vi "E7_20_READ_BUFFER.vi"(8 "error in":T6, 11 "DriverConnect in":T1={"InterfaceType"=enum."VISA", "OpenedSession"="", "InterfaceSettings"={"Interface"=enum."RS232", "EOS 4 read"=enum."LF (\\n)", "EOS 4 write"=enum."LF (\\n)", "TMO, ms"=10000, "Sett"=variant(cluster{"Baud Rate":u32, "Data Bits":u16, "Parity":u16, "Stop Bits":u16, "Flow Control":u16, "Eho":bool} {"Baud Rate"=75, "Data Bits"=0, "Parity"=0, "Stop Bits"=0, "Flow Control"=0, "Eho"=FALSE})}}) -> (0 "error out":T6, 3 "DriverConnect out":T1={"InterfaceType"=enum."VISA", "OpenedSession"="", "InterfaceSettings"={"Interface"=enum."RS232", "EOS 4 read"=enum."LF (\\n)", "EOS 4 write"=enum."LF (\\n)", "TMO, ms"=10000, "Sett"=variant(cluster{"Baud Rate":u32, "Data Bits":u16, "Parity":u16, "Stop Bits":u16, "Flow Control":u16, "Eho":bool} {"Baud Rate"=75, "Data Bits"=0, "Parity"=0, "Stop Bits"=0, "Flow Control"=0, "Eho"=FALSE})}}, 5 "String":string)   [LabVIEW 2018]
uses:
  MOKO_LabViewLibrary/MokoLowLevel/MokoLowLovelControl/MLLC_Error.ctl
  MOKO_LabViewLibrary/MokoLowLevel/MokoLowLovelControl/MLLC_ConnectCluster.ctl
  MOKO_LabViewLibrary/MokoLowLevel/MokoLowLovelControl/MLLC_InterfaceType.ctl
  MOKO_LabViewLibrary/MokoLowLevel/MokoLowLovelControl/MLLC_OpenedSession.ctl
  MOKO_LabViewLibrary/MokoLowLevel/MokoLowLovelControl/MLLC_InterfaceSettings.ctl
  MOKO_LabViewLibrary/MokoLowLevel/MokoLowLovelControl/MLLC_InterfaceKind.ctl
  MOKO_LabViewLibrary/MokoLowLevel/MokoLowLovelControl/MLLC_Rs232Settings.ctl
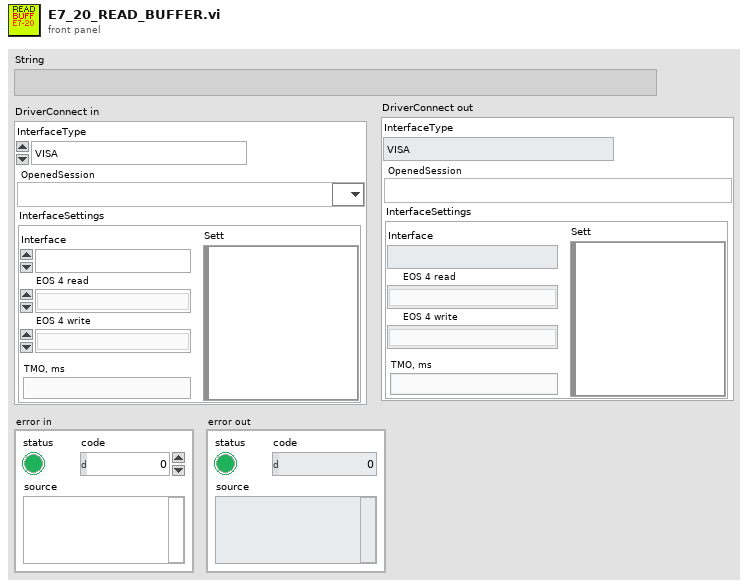
[diagram p1: front panel]
types:
  T1 = typedef "MLLC_ConnectCluster.ctl" = cluster{"InterfaceType":T2, "OpenedSession":T3, "InterfaceSettings":T4}
  T2 = typedef "MLLC_InterfaceType.ctl" = enum16{"VISA", "Prologix USB-GPIB"}
  T3 = typedef "MLLC_OpenedSession.ctl" = refnum<visa-resource-name>
  T4 = typedef "MLLC_InterfaceSettings.ctl" = cluster{"Interface":T5, "EOS 4 read":enum16{"Default (=EOS 4 write)", "CR (\\r)", "LF (\\n)", "None"}, "EOS 4 write":enum16{"CR+LF (\\r\\n)", "CR (\\r)", "LF (\\n)", "None"}, "TMO, ms":i32, "Sett":variant}
  T5 = typedef "MLLC_InterfaceKind.ctl" = enum16{"RS232", "GPIB", "USB", "Ethernet", "another"}
  T6 = typedef "MLLC_Error.ctl" = errorcluster
  T7 = typedef "MLLC_Rs232Settings.ctl" = cluster{"Baud Rate":u32, "Data Bits":u16, "Parity":u16, "Stop Bits":u16, "Flow Control":u16, "Eho":bool}
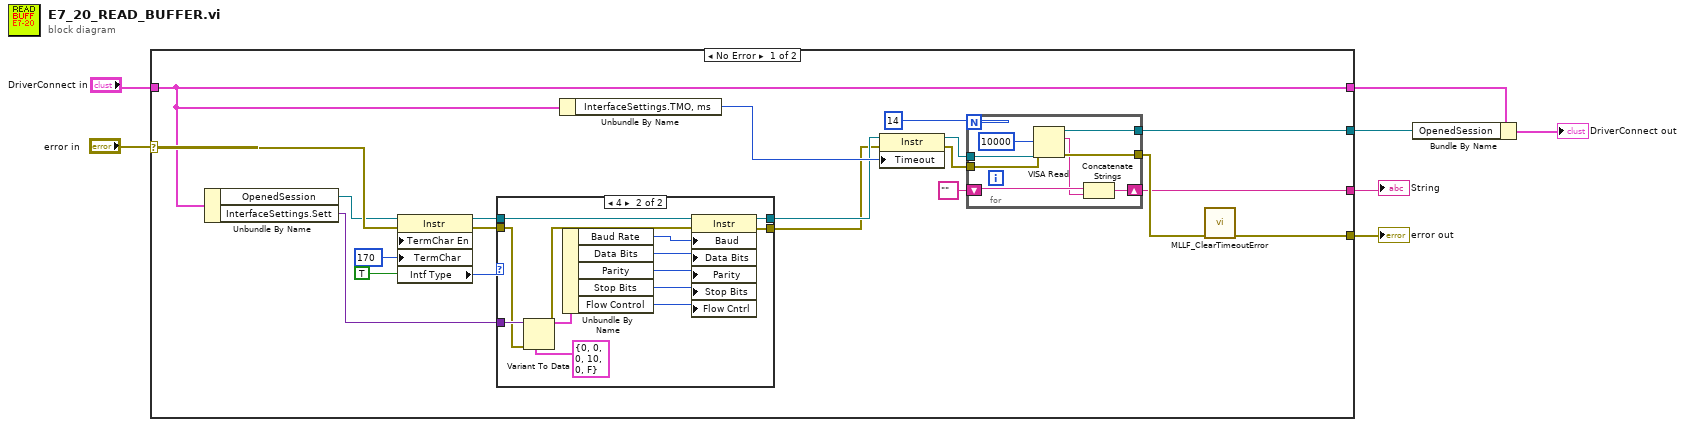
[diagram p0: block diagram]
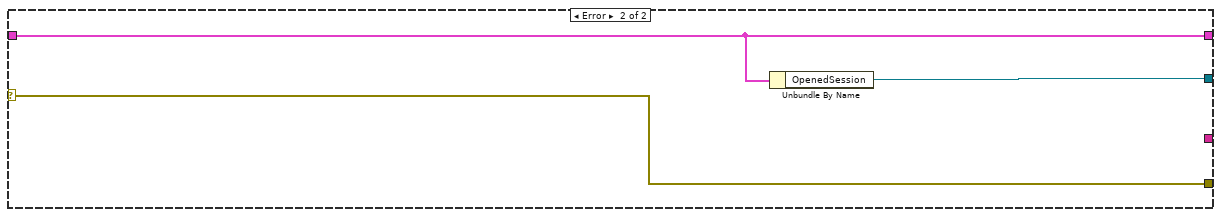
[diagram p3: hidden frame]
diagram:
  n1 = case shown="No Error" "error in" {
    selector: "error in" -> [w25 w53]
    tunnel: [w13 _] -> w7
    tunnel: [w27 w53] -> w6
    tunnel: [w14 w51] -> w3
    tunnel: [w9 w52] -> w2
    tunnel: "DriverConnect in" -> [w9 w52]
    frame No Error {
      n2 = Unbundle By Name(w9) -> ("OpenedSession"=w8:T3, "InterfaceSettings.Sett"=w22:variant)
      n3 = property class="Instr"(reference=w8, error in=w25, "TermChar En"=TRUE ("Message Based Settings:Termination Character Enable"), "TermChar"=u16 170 ("Message Based Settings:Termination Character")) -> (reference out=w24:T3, error out=w23:errorcluster, "Intf Type"=w18:u16)
      n4 = case shown="4" w18 {
        tunnel: [w37 w46] -> w19
        tunnel: w24 -> [w37 w47]
        tunnel: [w36 w38] -> w11
        tunnel: w23 -> [w36 w49]
        tunnel: w22 -> [_ w50]
        frame 0, Default {
        }
        frame 4 {
          n5 = Variant To Data(error in=w49, type=T7 {"Baud Rate"=0, "Data Bits"=0, "Parity"=0, "Stop Bits"=10, "Flow Control"=0, "Eho"=FALSE} ("Cluster"), Variant=w50) -> (data=w44:T7, error out=w48:errorcluster)
          n6 = Unbundle By Name(w44) -> ("Baud Rate"=w43:u32, "Data Bits"=w39:u16, "Parity"=w40:u16, "Stop Bits"=w41:u16, "Flow Control"=w42:u16)
          n7 = property class="Instr"(reference=w47, error in=w48, "Baud"=w43, "Data Bits"=w39, "Parity"=w40, "Stop Bits"=w41, "Flow Cntrl"=w42) -> (reference out=w46:T3, error out=w38:errorcluster)
        }
      }
      n8 = Unbundle By Name(w9) -> ("InterfaceSettings.TMO, ms"=w20:i32)
      n9 = property class="Instr"(reference=w19, error in=w11, "Timeout"=w20) -> (reference out=w17:T3, error out=w16:errorcluster)
      n10 = for {
        N: 14 ("length (rest)") -> [_]
        shift-right: [w30] -> w13
        shift-left: "" ("read buffer") -> [w29]
        tunnel: w17 -> [w34]
        tunnel: w16 -> [w33]
        tunnel: [w32] -> w15
        tunnel: [w31] -> w14
        n11 = VISA Read(VISA resource name=w34, byte count=u32 10000, error in (no error)=w33) -> (VISA resource name out=w31:T3, read buffer=w28:string, error out=w32:errorcluster)  [unwired: 1 out]
        n12 = Concatenate Strings(w29, w28) -> (w30:string)
      }
      n13 = call "MLLF_ClearTimeoutError.vi"("error in (no error)"=w15) -> ("error out"=w27:errorcluster)  [unwired: 10 in]
    }
    frame Error {
      n14 = Unbundle By Name(w52) -> ("OpenedSession"=w51:T3)
    }
  }
  "String" <- w7
  "error out" <- w6
  n15 = Bundle By Name(cluster=w2, "OpenedSession"=w3) -> (→"DriverConnect out":T1)
